vi "Test Write Date & Time.vi"(11 "TwinCAT ADS in":refnum<class "TwinCAT ADS.lvclass">) -> (3 "TwinCAT ADS out":refnum<class "TwinCAT ADS.lvclass">)   [LabVIEW 2018]
uses:
  TwinCAT ADS Class/TwinCAT ADS.lvclass
  1810e33a-9f28-4a9f-955d-88b2d52fcb7d.vi
  bddc9ca0-f439-4ec0-8378-2d656a15fdf5.vi
  6eb98df2-83f9-486c-9644-9c0be63e79d9.vi
  064d5dcb-7de0-49c5-9396-5bbe5b2bda3b.vi
  ee4c3017-c29e-4fe8-a368-edb52350add7.vi
  2b1c653c-d696-49ba-81e0-0abe759a7aaf.vi
  9eb3de2c-f32a-4594-b9ea-b097d7f01ba5.vi
  ec7047c1-9154-4949-a526-ee05bedf0e67.vi
  04b1d6c3-d363-4ba5-8c8b-88b588f9980c.vi
  96827efc-f82d-4e1c-9c1b-454960b395ec.vi
  7e66dc0a-1568-47cd-9851-5dc7b9fa6012.vi
  788e8c4b-cb26-40cd-92b4-362031163be5.vi
  58f04dc6-9466-4392-88d8-370a7d168ec8.vi
  7dc634db-efdd-42f4-a4b0-d96c414e946f.vi
  83d4cac9-4aba-4050-933e-bb2870508173.vi
  TwinCAT ADS Class/VIs/Data/Read.vi
  <vilib>/addons/_JKI Toolkits/Caraya/classes/Assert/Assert Equal Value and Type_Variant.vi
  <vilib>/addons/_JKI Toolkits/Caraya/classes/Assert/Assert.lvclass
  <vilib>/addons/_JKI Toolkits/Caraya/classes/Test/Test.lvclass
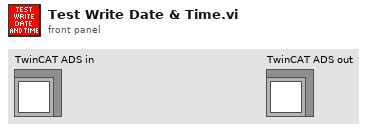
[diagram p1: front panel]
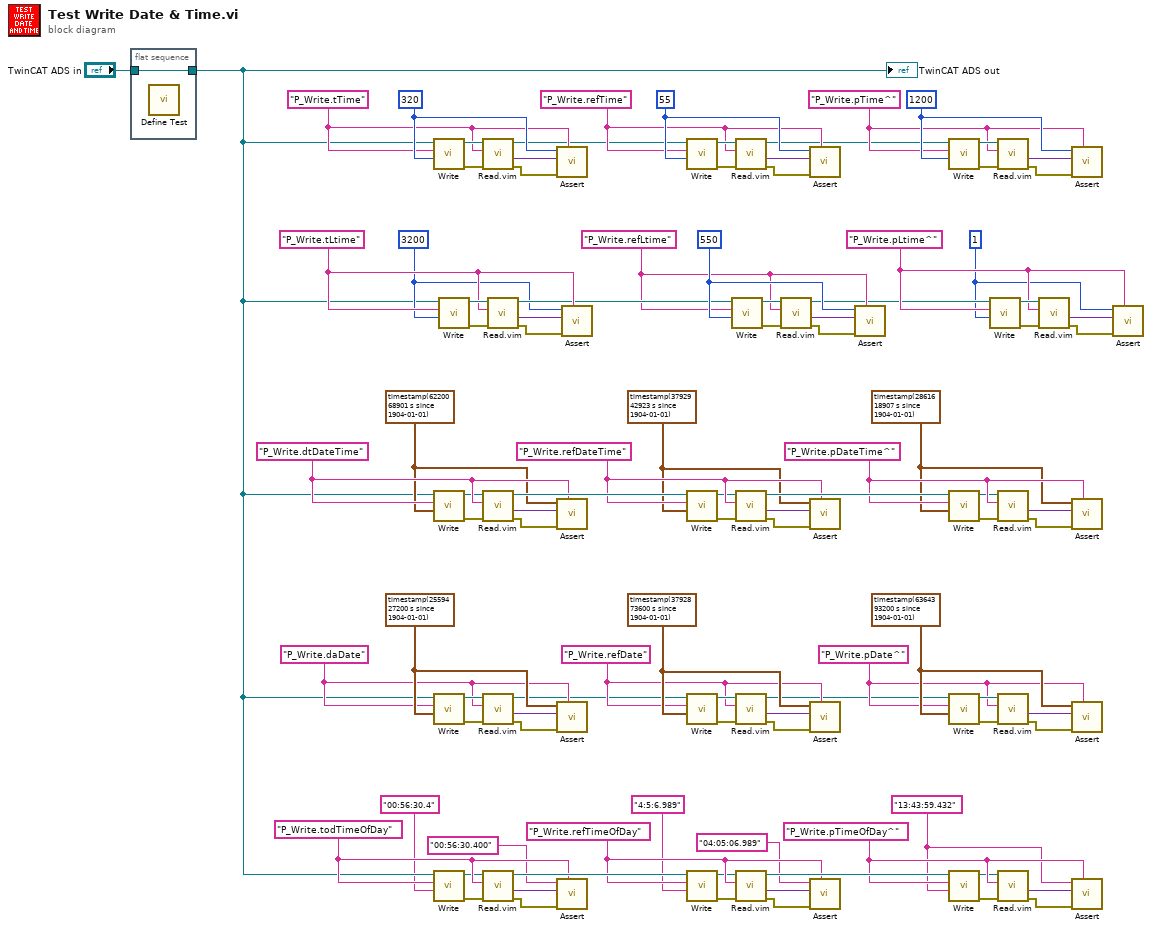
[diagram p0: block diagram]
diagram:
  w6 = "13:43:59.432" ("Symbol Name")
  w22 = "P_Write.pTimeOfDay^" ("Symbol Name")
  w17 = "P_Write.refTimeOfDay" ("Symbol Name")
  w13 = "P_Write.todTimeOfDay" ("Symbol Name")
  w43 = timestamp(6364393200 s since 1904-01-01) ("Value")
  w42 = timestamp(3792873600 s since 1904-01-01) ("Value")
  w40 = timestamp(2559427200 s since 1904-01-01) ("Value")
  w25 = "P_Write.pDate^" ("Symbol Name")
  w30 = "P_Write.refDate" ("Symbol Name")
  w35 = "P_Write.daDate" ("Symbol Name")
  w48 = u64 1 ("Value")
  w50 = "P_Write.pLtime^" ("Symbol Name")
  w44 = timestamp(2861618907 s since 1904-01-01) ("Value")
  w45 = timestamp(3792942923 s since 1904-01-01) ("Value")
  w54 = timestamp(6220068901 s since 1904-01-01) ("Value")
  w69 = "P_Write.pDateTime^" ("Symbol Name")
  w64 = "P_Write.refDateTime" ("Symbol Name")
  w59 = "P_Write.dtDateTime" ("Symbol Name")
  w71 = u64 3200 ("Value")
  w78 = u32 1200 ("Value")
  w73 = "P_Write.pTime^" ("Symbol Name")
  w81 = u64 550 ("Value")
  w79 = "P_Write.refLtime" ("Symbol Name")
  w88 = u32 55 ("Value")
  w87 = "P_Write.refTime" ("Symbol Name")
  w93 = "P_Write.tLtime" ("Symbol Name")
  w95 = u32 320 ("Value")
  w94 = "P_Write.tTime" ("Symbol Name")
  n1 = flat-sequence {
    tunnel: "TwinCAT ADS in" -> [w105]
    tunnel: [w105] -> w7
    frame #0 {
      n2 = call <vilib>:"Define Test.vi"() -> ()  [unwired: 10 in, 2 out]
    }
  }
  n3 = call "Write.vi"("Value"=w95, "Symbol Name"=w94, "TwinCAT ADS in"=w7) -> ("error out"=w102:errorcluster, "TwinCAT ADS out"=w103:refnum<class "TwinCAT ADS.lvclass">)  [unwired: 7 in]
  n4 = call "Write.vi"("Value"=w54, "Symbol Name"=w59, "TwinCAT ADS in"=w7) -> ("error out"=w56:errorcluster, "TwinCAT ADS out"=w55:refnum<class "TwinCAT ADS.lvclass">)  [unwired: 7 in]
  n5 = call "Write.vi"("Value"=w40, "Symbol Name"=w35, "TwinCAT ADS in"=w7) -> ("error out"=w38:errorcluster, "TwinCAT ADS out"=w39:refnum<class "TwinCAT ADS.lvclass">)  [unwired: 7 in]
  n6 = call "Write.vi"("Value"="00:56:30.4" ("Symbol Name"), "Symbol Name"=w13, "TwinCAT ADS in"=w7) -> ("error out"=w10:errorcluster, "TwinCAT ADS out"=w9:refnum<class "TwinCAT ADS.lvclass">)  [unwired: 7 in]
  n7 = call "Write.vi"("Value"=w71, "Symbol Name"=w93, "TwinCAT ADS in"=w7) -> ("error out"=w97:errorcluster, "TwinCAT ADS out"=w96:refnum<class "TwinCAT ADS.lvclass">)  [unwired: 7 in]
  n8 = call "Read.vim"("error in (no error)"=w102, "Symbol Name"=w94, "TwinCAT ADS in"=w103) -> ("error out"=w101:errorcluster, "Value"=w100:variant, "TwinCAT ADS out"=w86:refnum<class "TwinCAT ADS.lvclass">)  [unwired: 6 in]
  n9 = call "Read.vim"("error in (no error)"=w56, "Symbol Name"=w59, "TwinCAT ADS in"=w55) -> ("error out"=w57:errorcluster, "Value"=w58:variant, "TwinCAT ADS out"=w65:refnum<class "TwinCAT ADS.lvclass">)  [unwired: 6 in]
  n10 = call "Read.vim"("error in (no error)"=w38, "Symbol Name"=w35, "TwinCAT ADS in"=w39) -> ("error out"=w37:errorcluster, "Value"=w36:variant, "TwinCAT ADS out"=w29:refnum<class "TwinCAT ADS.lvclass">)  [unwired: 6 in]
  n11 = call "Read.vim"("error in (no error)"=w10, "Symbol Name"=w13, "TwinCAT ADS in"=w9) -> ("error out"=w11:errorcluster, "Value"=w12:variant, "TwinCAT ADS out"=w18:refnum<class "TwinCAT ADS.lvclass">)  [unwired: 6 in]
  n12 = call "Read.vim"("error in (no error)"=w97, "Symbol Name"=w93, "TwinCAT ADS in"=w96) -> ("error out"=w98:errorcluster, "Value"=w99:variant, "TwinCAT ADS out"=w80:refnum<class "TwinCAT ADS.lvclass">)  [unwired: 6 in]
  n13 = call-poly <vilib>:"Assert.vi"("Label"=w94, "error in (no error)"=w101, "Y"=w100, "X"=w95) -> ()  [unwired: 6 in, 2 out]
  n14 = call-poly <vilib>:"Assert.vi"("Label"=w59, "error in (no error)"=w57, "Y"=w58, "X"=w54) -> ()  [unwired: 6 in, 2 out]
  n15 = call-poly <vilib>:"Assert.vi"("Label"=w35, "error in (no error)"=w37, "Y"=w36, "X"=w40) -> ()  [unwired: 6 in, 2 out]
  n16 = call-poly <vilib>:"Assert.vi"("Label"=w13, "error in (no error)"=w11, "Y"=w12, "X"="00:56:30.400" ("Symbol Name")) -> ()  [unwired: 6 in, 2 out]
  n17 = call-poly <vilib>:"Assert.vi"("Label"=w93, "error in (no error)"=w98, "Y"=w99, "X"=w71) -> ()  [unwired: 6 in, 2 out]
  n18 = call "Write.vi"("Value"=w88, "Symbol Name"=w87, "TwinCAT ADS in"=w86) -> ("error out"=w91:errorcluster, "TwinCAT ADS out"=w92:refnum<class "TwinCAT ADS.lvclass">)  [unwired: 7 in]
  n19 = call "Write.vi"("Value"=w45, "Symbol Name"=w64, "TwinCAT ADS in"=w65) -> ("error out"=w61:errorcluster, "TwinCAT ADS out"=w60:refnum<class "TwinCAT ADS.lvclass">)  [unwired: 7 in]
  n20 = call "Write.vi"("Value"=w42, "Symbol Name"=w30, "TwinCAT ADS in"=w29) -> ("error out"=w33:errorcluster, "TwinCAT ADS out"=w34:refnum<class "TwinCAT ADS.lvclass">)  [unwired: 7 in]
  n21 = call "Write.vi"("Value"="4:5:6.989" ("Symbol Name"), "Symbol Name"=w17, "TwinCAT ADS in"=w18) -> ("error out"=w15:errorcluster, "TwinCAT ADS out"=w14:refnum<class "TwinCAT ADS.lvclass">)  [unwired: 7 in]
  n22 = call "Write.vi"("Value"=w81, "Symbol Name"=w79, "TwinCAT ADS in"=w80) -> ("error out"=w84:errorcluster, "TwinCAT ADS out"=w85:refnum<class "TwinCAT ADS.lvclass">)  [unwired: 7 in]
  n23 = call "Read.vim"("error in (no error)"=w91, "Symbol Name"=w87, "TwinCAT ADS in"=w92) -> ("error out"=w90:errorcluster, "Value"=w89:variant, "TwinCAT ADS out"=w72:refnum<class "TwinCAT ADS.lvclass">)  [unwired: 6 in]
  n24 = call "Read.vim"("error in (no error)"=w61, "Symbol Name"=w64, "TwinCAT ADS in"=w60) -> ("error out"=w62:errorcluster, "Value"=w63:variant, "TwinCAT ADS out"=w70:refnum<class "TwinCAT ADS.lvclass">)  [unwired: 6 in]
  n25 = call "Read.vim"("error in (no error)"=w33, "Symbol Name"=w30, "TwinCAT ADS in"=w34) -> ("error out"=w32:errorcluster, "Value"=w31:variant, "TwinCAT ADS out"=w24:refnum<class "TwinCAT ADS.lvclass">)  [unwired: 6 in]
  n26 = call "Read.vim"("error in (no error)"=w15, "Symbol Name"=w17, "TwinCAT ADS in"=w14) -> ("error out"=w16:errorcluster, "Value"=w2:variant, "TwinCAT ADS out"=w23:refnum<class "TwinCAT ADS.lvclass">)  [unwired: 6 in]
  n27 = call "Read.vim"("error in (no error)"=w84, "Symbol Name"=w79, "TwinCAT ADS in"=w85) -> ("error out"=w83:errorcluster, "Value"=w82:variant, "TwinCAT ADS out"=w49:refnum<class "TwinCAT ADS.lvclass">)  [unwired: 6 in]
  n28 = call-poly <vilib>:"Assert.vi"("Label"=w87, "error in (no error)"=w90, "Y"=w89, "X"=w88) -> ()  [unwired: 6 in, 2 out]
  n29 = call-poly <vilib>:"Assert.vi"("Label"=w64, "error in (no error)"=w62, "Y"=w63, "X"=w45) -> ()  [unwired: 6 in, 2 out]
  n30 = call-poly <vilib>:"Assert.vi"("Label"=w30, "error in (no error)"=w32, "Y"=w31, "X"=w42) -> ()  [unwired: 6 in, 2 out]
  n31 = call-poly <vilib>:"Assert.vi"("Label"=w17, "error in (no error)"=w16, "Y"=w2, "X"="04:05:06.989" ("Symbol Name")) -> ()  [unwired: 6 in, 2 out]
  n32 = call-poly <vilib>:"Assert.vi"("Label"=w79, "error in (no error)"=w83, "Y"=w82, "X"=w81) -> ()  [unwired: 6 in, 2 out]
  n33 = call "Write.vi"("Value"=w78, "Symbol Name"=w73, "TwinCAT ADS in"=w72) -> ("error out"=w75:errorcluster, "TwinCAT ADS out"=w74:refnum<class "TwinCAT ADS.lvclass">)  [unwired: 7 in]
  n34 = call "Write.vi"("Value"=w44, "Symbol Name"=w69, "TwinCAT ADS in"=w70) -> ("error out"=w67:errorcluster, "TwinCAT ADS out"=w68:refnum<class "TwinCAT ADS.lvclass">)  [unwired: 7 in]
  n35 = call "Write.vi"("Value"=w43, "Symbol Name"=w25, "TwinCAT ADS in"=w24) -> ("error out"=w27:errorcluster, "TwinCAT ADS out"=w26:refnum<class "TwinCAT ADS.lvclass">)  [unwired: 7 in]
  n36 = call "Write.vi"("Value"=w6, "Symbol Name"=w22, "TwinCAT ADS in"=w23) -> ("error out"=w20:errorcluster, "TwinCAT ADS out"=w21:refnum<class "TwinCAT ADS.lvclass">)  [unwired: 7 in]
  n37 = call "Write.vi"("Value"=w48, "Symbol Name"=w50, "TwinCAT ADS in"=w49) -> ("error out"=w52:errorcluster, "TwinCAT ADS out"=w51:refnum<class "TwinCAT ADS.lvclass">)  [unwired: 7 in]
  n38 = call "Read.vim"("error in (no error)"=w75, "Symbol Name"=w73, "TwinCAT ADS in"=w74) -> ("error out"=w76:errorcluster, "Value"=w77:variant)  [unwired: 6 in, 1 out]
  n39 = call "Read.vim"("error in (no error)"=w67, "Symbol Name"=w69, "TwinCAT ADS in"=w68) -> ("error out"=w66:errorcluster, "Value"=w46:variant)  [unwired: 6 in, 1 out]
  n40 = call "Read.vim"("error in (no error)"=w27, "Symbol Name"=w25, "TwinCAT ADS in"=w26) -> ("error out"=w28:errorcluster, "Value"=w41:variant)  [unwired: 6 in, 1 out]
  n41 = call "Read.vim"("error in (no error)"=w20, "Symbol Name"=w22, "TwinCAT ADS in"=w21) -> ("error out"=w19:errorcluster, "Value"=w8:variant)  [unwired: 6 in, 1 out]
  n42 = call "Read.vim"("error in (no error)"=w52, "Symbol Name"=w50, "TwinCAT ADS in"=w51) -> ("error out"=w53:errorcluster, "Value"=w47:variant)  [unwired: 6 in, 1 out]
  n43 = call-poly <vilib>:"Assert.vi"("Label"=w73, "error in (no error)"=w76, "Y"=w77, "X"=w78) -> ()  [unwired: 6 in, 2 out]
  n44 = call-poly <vilib>:"Assert.vi"("Label"=w69, "error in (no error)"=w66, "Y"=w46, "X"=w44) -> ()  [unwired: 6 in, 2 out]
  n45 = call-poly <vilib>:"Assert.vi"("Label"=w25, "error in (no error)"=w28, "Y"=w41, "X"=w43) -> ()  [unwired: 6 in, 2 out]
  n46 = call-poly <vilib>:"Assert.vi"("Label"=w22, "error in (no error)"=w19, "Y"=w8, "X"=w6) -> ()  [unwired: 6 in, 2 out]
  n47 = call-poly <vilib>:"Assert.vi"("Label"=w50, "error in (no error)"=w53, "Y"=w47, "X"=w48) -> ()  [unwired: 6 in, 2 out]
  "TwinCAT ADS out" <- w7
